vi "Get SDO Response.vi"(11 "CANopen in":refnum<class "CANopen.lvclass">) -> (2 "SDO Response":refnum<notifier>, 3 "CANopen out":refnum<class "CANopen.lvclass">)   [LabVIEW 2024, in "canopen.lvlib" / "CANopen.lvclass"]
uses:
  CANopen.lvclass
  CANopen.lvclass/CANopen.ctl
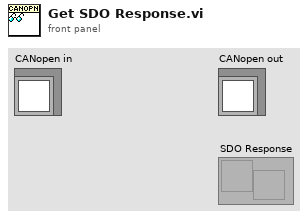
[diagram p1: front panel]
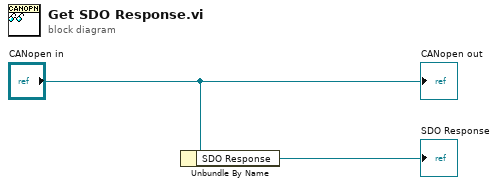
[diagram p0: block diagram]
diagram:
  n1 = Unbundle By Name("CANopen in") -> ("SDO Response"=→"SDO Response":refnum<notifier>)
  "CANopen out" <- "CANopen in"
